vi "Trigger Control.vi"(8 "Invert?":bool, 10 "Axis 2 In":dbl, 11 "Axis 1 In":dbl) -> (3 "Axis Out":dbl)   [LabVIEW 2016]
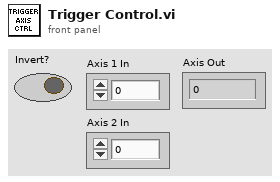
[diagram p1: front panel]
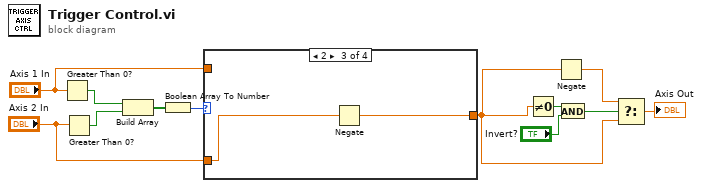
[diagram p0: block diagram]
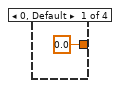
[diagram p2: hidden frame]
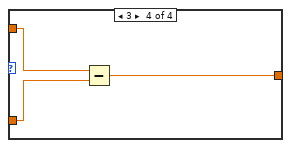
[diagram p4: hidden frame]
diagram:
  n1 = Greater Than 0?(x="Axis 1 In") -> (x > 0?=w12:bool)
  n2 = Greater Than 0?(x="Axis 2 In") -> (x > 0?=w11:bool)
  n3 = Build Array(w12, w11) -> (w10:bool[])
  n4 = Boolean Array To Number(Boolean array=w10) -> (number=w9:u32)
  n5 = case shown="2" w9 {
    tunnel: "Axis 1 In" -> [_ w14 _ w19]
    tunnel: "Axis 2 In" -> [_ _ w16 w18]
    tunnel: [0.0 w14 w15 w17] -> w3
    frame 0, Default {
    }
    frame 1 {
    }
    frame 2 {
      n6 = Negate(x=w16) -> (-x=w15:dbl)
    }
    frame 3 {
      n7 = Subtract(x=w19, y=w18) -> (x-y=w17:dbl)
    }
  }
  n8 = Not Equal To 0?(x=w3) -> (x != 0?=w4:bool)
  n9 = Negate(x=w3) -> (-x=w2:dbl)
  n10 = And(x=w4, y="Invert?") -> (x .and. y?=w5:bool)
  n11 = Select(t=w2, s=w5, f=w3) -> (s? t:f=→"Axis Out":dbl)
